vi "main.vi"() -> ()   [LabVIEW 2020]
doc: "This VI simulates the heat propagation and in/out flow in a square tank.\n\nThe heat propagation model used is a 2D rectangular heat wave PDE model to approximate the propagation of the heat in the liquid inside the tank. A heater is considered at the center of the base of the tank with set width and controllable output power. The walls of the tank are considered perfectly isolated. The heat losses are calculated by conduction from the surface of the liquid, through the air, to the outside (at room temperature).\n\nThe volume flow is controlled through the matrix that simulates the liquid for the PDE, that is, when enough volume is to be added to the tank, we add another row of points to the simulation (resp. remove for outward flow). Liquid is added at room temperature at the surface and removed from the bottom.\n\nThe transducers and actuators are modelled in this VI in such a way that the On/Off controller for the temperature (between EH 01 and TI 05) simulates a controller in a real plant. Room temperature is the only not-sensed-nor-actuated available variable to be used as noise. The tank graph should not be visible as well, but it makes the simulation much more pleasant to the eyes."
uses:
  TankResolution.ctl
  Heater.ctl
  <vilib>/Utility/error.llb/DialogType.ctl
panel:
  in  "temp_set_point":dbl(slide)=298.15 scale=0.0..100.0
  in  "temp_control":bool
  out "level_show":dbl format="%_3g m"
  out "temp_show_05":dbl format="%_3g ºC"
  out "temp_show_04":dbl format="%_3g ºC"
  out "temp_show_03":dbl format="%_3g ºC"
  out "temp_show_02":dbl format="%_3g ºC"
  out "temp_show_01":dbl format="%_3g ºC"
  out "termometer_05":dbl(slide) scale=0.0..100.0
  out "termometer_04":dbl(slide) scale=0.0..100.0
  out "termometer_03":dbl(slide) scale=0.0..100.0
  out "termometer_02":dbl(slide) scale=0.0..100.0
  out "termometer_01":dbl(slide) scale=0.0..100.0
  in  "BV 02":dbl(knob) scale=0.0..5.0
  in  "BV 01":dbl(knob) scale=0.0..5.0
  in  "EH 01":bool
  out "LI 01":dbl
  out "water_level":dbl
  out "TI 05":dbl
  out "TI 04":dbl
  out "TI 03":dbl
  out "TI 02":dbl
  out "TI 01":dbl
  out "temp_5":dbl
  out "temp_4":dbl
  out "temp_3":dbl
  out "temp_2":dbl
  out "temp_1":dbl
  out "out_flow (m^3/s)":dbl(knob) min=0.0 max=0.5 scale=0.0..0.01
  out "in_flow (m^3/s)":dbl(knob) min=0.0 max=0.5 scale=0.0..0.01
  in  "room_temperature":dbl(slide)=298.15 scale=273.15..373.15
  in  "heater":dbl(knob) scale=0.0..50.0
  in  "stop":bool
  out "PDE Plot":dbl[][](graph)
  # "Tank Model"
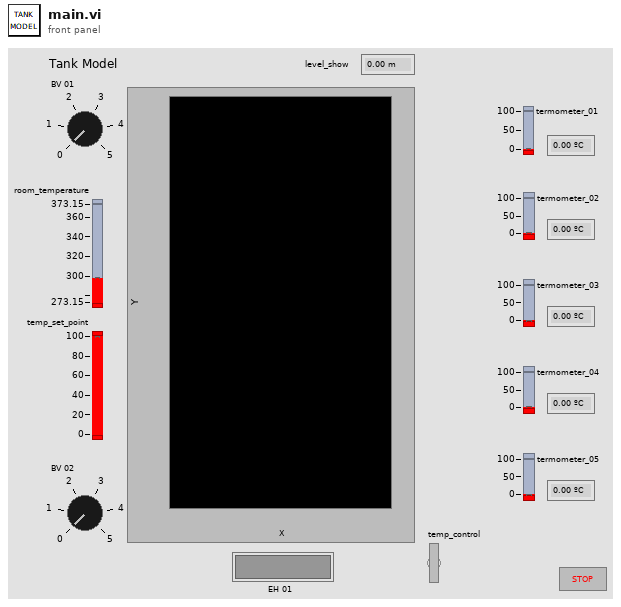
[diagram p1: front panel]
types:
  T1 = typedef "TankResolution.ctl" = cluster{"y_points_per_meter":i32, "x_points_per_meter":i32, "n_t_points":i32, "tank_height":dbl, "tank_width":dbl, "t_length_ms":u32}
  T2 = typedef "Liquid.ctl" = cluster{"liquid_temperature":dbl[][], "water_level":dbl, "room_temperature":dbl}
  T3 = typedef "DialogType.ctl" = u16
  T4 = typedef "Heater.ctl" = cluster{"heater_width":dbl, "heater_heat":dbl}
  T5 = typedef "LVOffsetAndMultiplierTypeDef.ctl" = cluster{"Offset":dbl, "Multiplier":dbl}
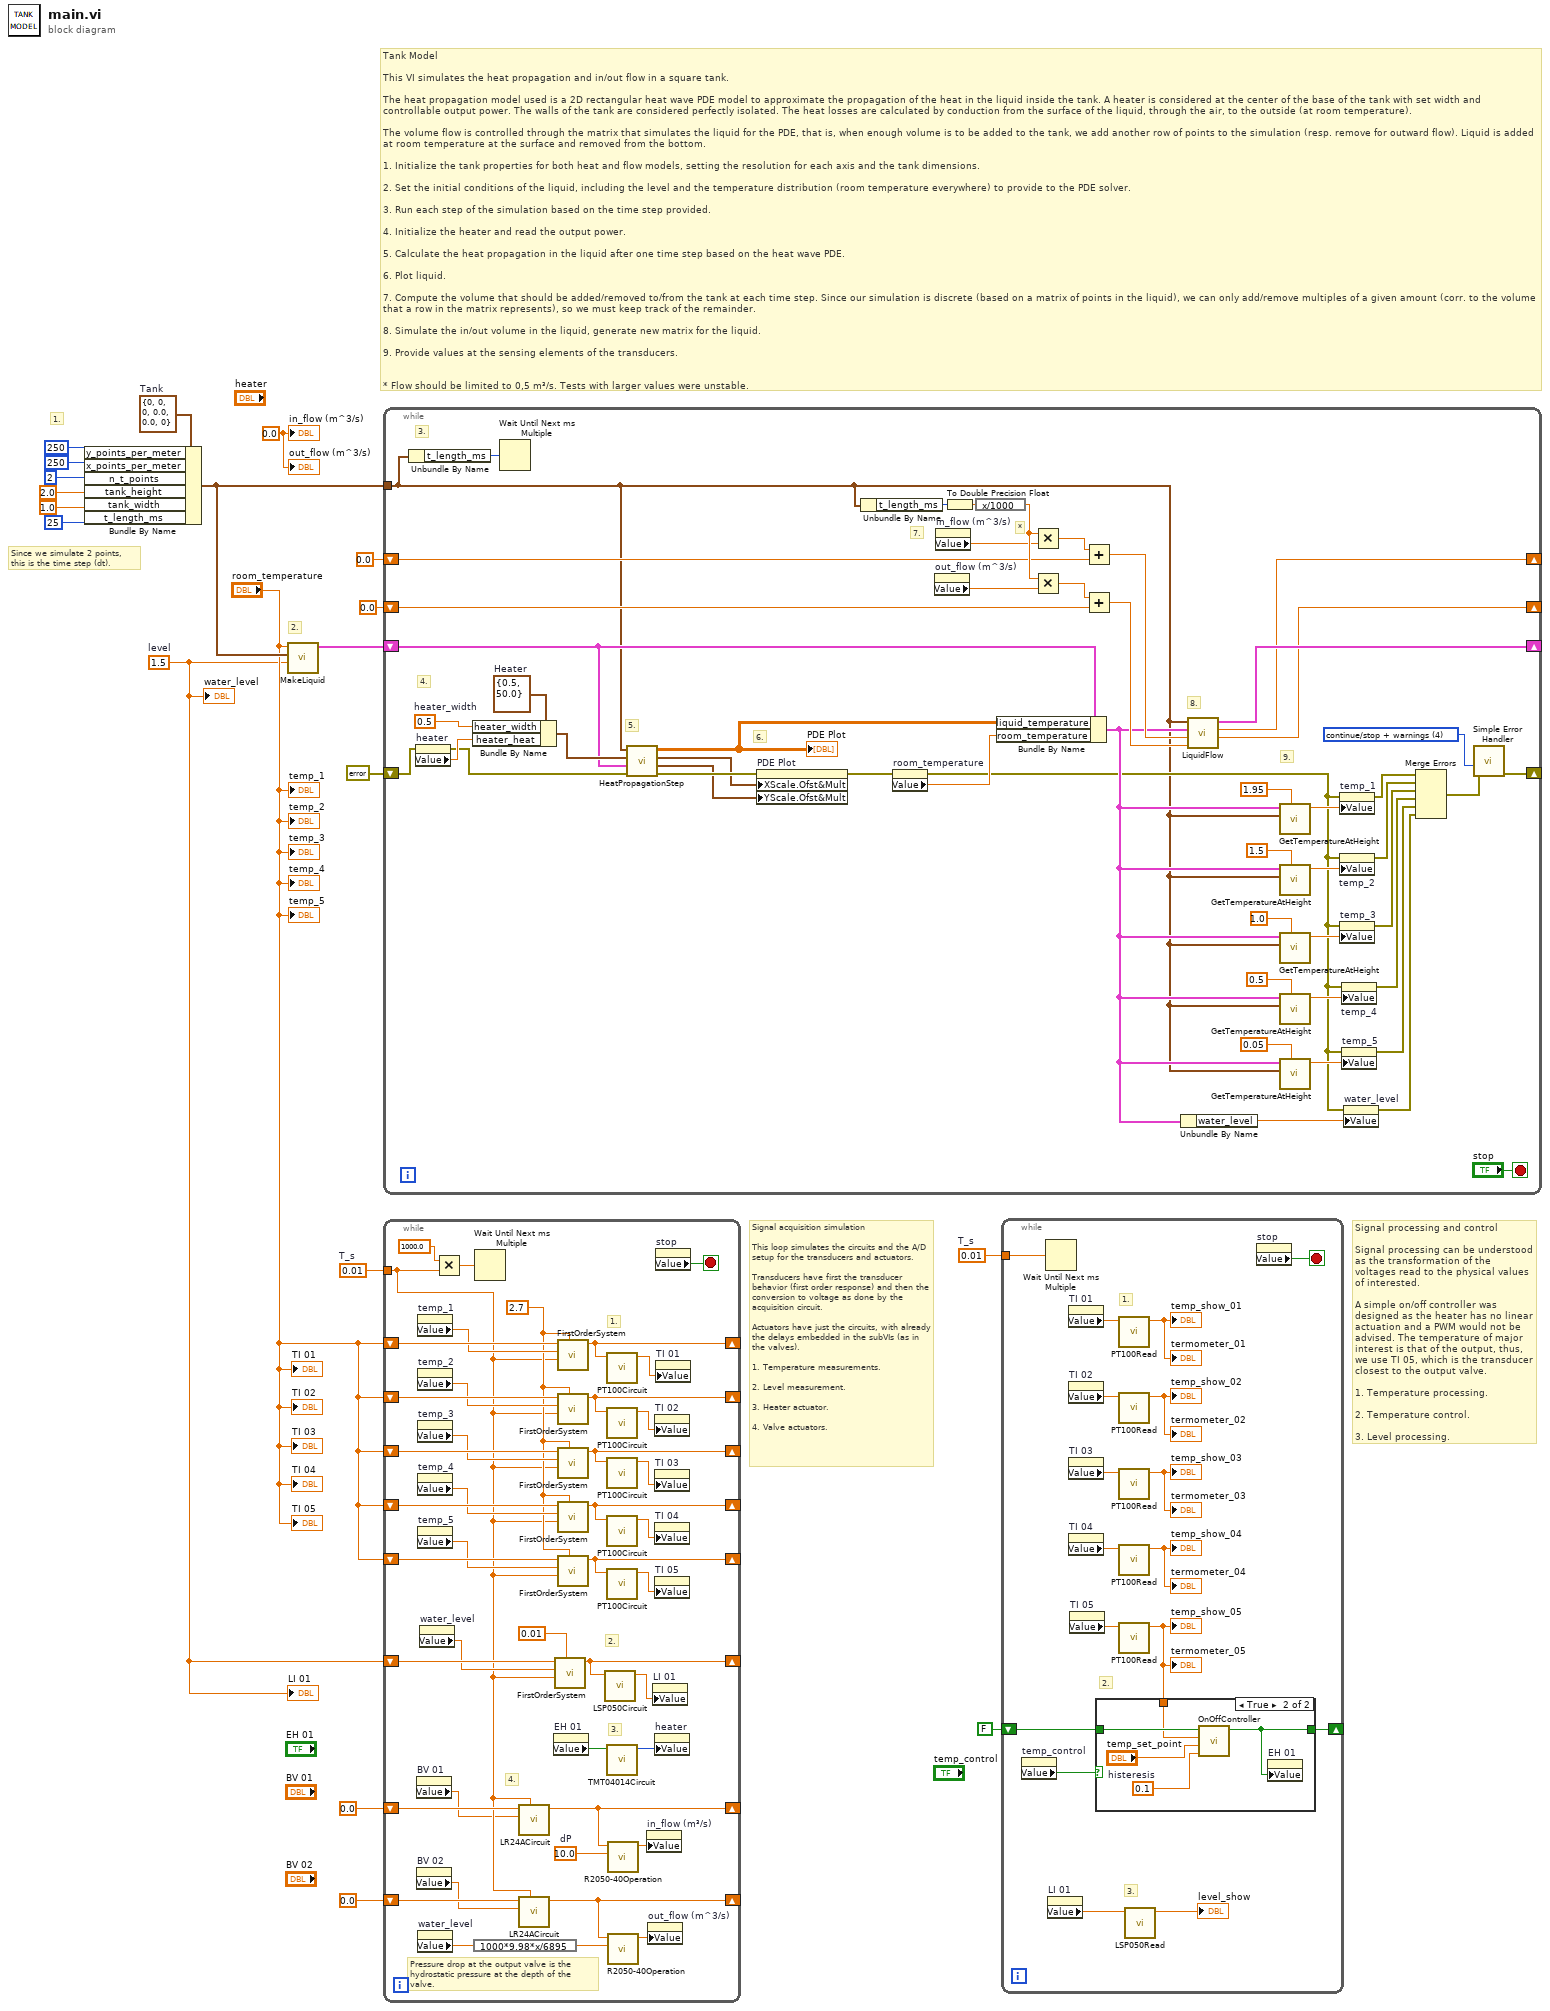
[diagram p0: block diagram]
diagram:
  w2 = 0.01  # T_s
  w5 = 0.0 ("in_flow (m")
  w8 = 0.01  # T_s
  w6 = 1.5  # level
  w20 = T1 {"y_points_per_meter"=0, "x_points_per_meter"=0, "n_t_points"=0, "tank_height"=0.0, "tank_width"=0.0, "t_length_ms"=0}  # Tank
  # "Signal processing and control\n\nSignal processing can be understood as the transformation of the voltages read to the physical values of interested.\n\nA simple on/off controller was designed as the heater has no linear actuation and a PWM would not be advised. The temperature of major interest is that of the output, thus, we use TI 05, which is the transducer closest to the output valve.\n\n1. Temperature processing.\n\n2. Temperature control.\n\n3. Level processing."
  # "Signal acquisition simulation\n\nThis loop simulates the circuits and the A/D setup for the transducers and actuators.\n\nTransducers have first the transducer behavior (first order response) and then the conversion to voltage as done by the acquisition circuit.\n\nActuators have just the circuits, with already the delays embedded in the subVIs (as in the valves).\n\n1. Temperature measurements.\n\n2. Level measurement.\n\n3. Heater actuator.\n\n4. Valve actuators."
  # "1."
  # "Tank Model\n\nThis VI simulates the heat propagation and in/out flow in a square tank.\n\nThe heat propagation model used is a 2D rectangular heat wave PDE model to approximate the propagation of the heat in the liquid inside the tank. A heater is considered at the center of the base of the tank with set width and controllable output power. The walls of the tank are considered perfectly isolated. The heat losses are calculated by conduction from the surface of the liquid, through the air, to the outside (at room temperature).\n\nThe volume flow is controlled through the matrix that simulates the liquid for the PDE, that is, when enough volume is to be added to the tank, we add another row of points to the simulation (resp. remove for outward flow). Liquid is added at room temperature at the surface and removed from the bottom.\n\n1. Initialize the tank properties for both heat and flow models, setting the resolution for each axis and the tank dimensions.\n\n2. Set the initial conditions of the liquid, including the level and the temperature distribution (room temperature everywhere) to provide to the PDE solver.\n\n3. Run each step of the simulation based on the time step provided.\n\n4. Initialize the heater and read the output power.\n\n5. Calculate the heat propagation in the liquid after one time step based on the heat wave PDE.\n\n6. Plot liquid.\n\n7. Compute the volume that should be added/removed to/from the tank at each time step. Since our simulation is discrete (based on a matrix of points in the liquid), we can only add/remove multiples of a given amount (corr. to the volume that a row in the matrix represents), so we must keep track of the remainder.\n\n8. Simulate the in/out volume in the liquid, generate new matrix for the liquid.\n\n9. Provide values at the sensing elements of the transducers.\n\n\n* Flow should be limited to 0,5 m³/s. Tests with larger values were unstable."
  # "2."
  # "Since we simulate 2 points,\nthis is the time step (dt)."
  n1 = Bundle By Name(cluster=w20, "y_points_per_meter"=250 ("n_y_points"), "x_points_per_meter"=250 ("x_resolution"), "n_t_points"=2, "tank_height"=2.0 ("y_length"), "tank_width"=1.0 ("x_length"), "t_length_ms"=u32 25) -> (w13:T1)
  n2 = call "MakeLiquid.vi"("level"=w6, "tank"=w13, "room_temperature"="room_temperature") -> ("liquid"=w12:T2)  [unwired: 8 in]
  n3 = while {
    tunnel: w13 -> [w21]
    shift-right: [w55] -> _
    shift-left: errorcluster {"status"=FALSE, "code"=0, "source"=""} ("error out") -> [w25]
    shift-right: [w50] -> _
    shift-left: w12 -> [w53]
    shift-right: [w49] -> _
    shift-left: 0.0 ("cumm_in_flow") -> [w56]
    shift-right: [w48] -> _
    shift-left: 0.0 ("cumm_out_flow") -> [w57]
    stop <- "stop" stop-if-true
    w54 = T3 4 items=["no dialog", "OK message", "continue or stop message", "OK message + warnings", "continue/stop + warnings"] ("type of dialog (OK msg:1)")
    w67 = T4 {"heater_width"=0.5, "heater_heat"=50.0}  # Heater
    w68 = 0.5  # heater_width
    # "9."
    # "*"
    # "6."
    # "4."
    # "3."
    # "8."
    # "7."
    # "5."
    n4 = Unbundle By Name(w21) -> ("t_length_ms"=w58:u32)
    n5 = property on="heater" class="Knob (strict)"(error in=w25) -> (error out=w24:errorcluster, "Value"=w26:dbl)  [unwired: 1 in, 1 out]
    n6 = Bundle By Name(cluster=w67, "heater_width"=w68, "heater_heat"=w26) -> (w66:T4)
    n7 = Wait Until Next ms Multiple(millisecond multiple=w58) -> ()  [unwired: 1 out]
    n8 = call "HeatPropagationStep.vi"("error in (no error)"=w24, "liquid"=w53, "heater"=w66, "tank"=w21) -> ("error out"=w72:errorcluster, "Y Scale"=w70:T5, "X Scale"=w71:T5, "next_temperature"=w47:dbl[][])  [unwired: 3 in]
    "PDE Plot" <- w47
    n9 = property on="PDE Plot" class="IntGraph (strict)"(error in=w72, "XScale.Ofst&Mult"=w71, "YScale.Ofst&Mult"=w70) -> (error out=w65:errorcluster)  [unwired: 1 in, 1 out]
    n10 = Unbundle By Name(w21) -> ("t_length_ms"=w59:u32)
    n11 = property on="room_temperature" class="Slide (strict)"(error in=w65) -> (error out=w27:errorcluster, "Value"=w64:dbl)  [unwired: 1 in, 1 out]
    n12 = property on="out_flow (m^3/s)" class="Knob (strict)"() -> ("Value"=w22:dbl)  [unwired: 2 in, 2 out]
    n13 = property on="in_flow (m^3/s)" class="Knob (strict)"() -> ("Value"=w23:dbl)  [unwired: 2 in, 2 out]
    n14 = To Double Precision Float(number=w59) -> (double precision float=w60:dbl)
    n15 = expression code="x/1000"(w60) -> (w63:dbl)
    n16 = Bundle By Name(cluster=w53, "liquid_temperature"=w47, "room_temperature"=w64) -> (w30:T2)
    n17 = Multiply(x=w63, y=w23) -> (x*y=w62:dbl)
    n18 = Multiply(x=w63, y=w22) -> (x*y=w61:dbl)
    n19 = Add(x=w62, y=w56) -> (x+y=w52:dbl)
    n20 = Add(x=w61, y=w57) -> (x+y=w51:dbl)
    n21 = Unbundle By Name(w30) -> ("water_level"=w29:dbl)
    n22 = call "LiquidFlow.vi"("out_vol"=w51, "in_vol"=w52, "liquid"=w30, "tank"=w21) -> ("remainder_out_vol"=w48:dbl, "remainder_in_vol"=w49:dbl, "next_liquid"=w50:T2)  [unwired: 5 in]
    n23 = call "GetTemperatureAtHeight.vi"("height"=1.95 ("tank_height"), "tank"=w21, "liquid"=w30) -> ("temperature"=w46:dbl)  [unwired: 8 in]
    n24 = call "GetTemperatureAtHeight.vi"("height"=1.5 ("tank_height"), "tank"=w21, "liquid"=w30) -> ("temperature"=w37:dbl)  [unwired: 8 in]
    n25 = call "GetTemperatureAtHeight.vi"("height"=1.0 ("tank_height"), "tank"=w21, "liquid"=w30) -> ("temperature"=w38:dbl)  [unwired: 8 in]
    n26 = call "GetTemperatureAtHeight.vi"("height"=0.5 ("tank_height"), "tank"=w21, "liquid"=w30) -> ("temperature"=w39:dbl)  [unwired: 8 in]
    n27 = call "GetTemperatureAtHeight.vi"("height"=0.05 ("tank_height"), "tank"=w21, "liquid"=w30) -> ("temperature"=w40:dbl)  [unwired: 8 in]
    n28 = property on="temp_1" class="DigNum (strict)"(error in=w27, "Value"=w46) -> (error out=w35:errorcluster)  [unwired: 1 in, 1 out]
    n29 = property on="temp_2" class="DigNum (strict)"(error in=w27, "Value"=w37) -> (error out=w34:errorcluster)  [unwired: 1 in, 1 out]
    n30 = property on="temp_3" class="DigNum (strict)"(error in=w27, "Value"=w38) -> (error out=w32:errorcluster)  [unwired: 1 in, 1 out]
    n31 = property on="temp_4" class="DigNum (strict)"(error in=w27, "Value"=w39) -> (error out=w31:errorcluster)  [unwired: 1 in, 1 out]
    n32 = property on="temp_5" class="DigNum (strict)"(error in=w27, "Value"=w40) -> (error out=w33:errorcluster)  [unwired: 1 in, 1 out]
    n33 = property on="water_level" class="DigNum (strict)"(error in=w27, "Value"=w29) -> (error out=w28:errorcluster)  [unwired: 1 in, 1 out]
    n34 = Merge Errors(w35, w34, w32, w31, w33, w28) -> (w36:errorcluster)
    n35 = call <vilib>:"Simple Error Handler.vi"("type of dialog (OK msg:1)"=w54, "error in (no error)"=w36) -> ("error out"=w55:errorcluster)  [unwired: 3 in, 4 out]
  }
  n36 = while {
    tunnel: w8 -> [w81]
    shift-right: [w101] -> _
    shift-left: "room_temperature" -> [w114]
    shift-right: [w99] -> _
    shift-left: "room_temperature" -> [w111]
    shift-right: [w98] -> _
    shift-left: "room_temperature" -> [w112]
    shift-right: [w97] -> _
    shift-left: "room_temperature" -> [w110]
    shift-right: [w96] -> _
    shift-left: "room_temperature" -> [w109]
    shift-right: [w88] -> _
    shift-left: w6 -> [w91]
    shift-right: [w83] -> _
    shift-left: 0.0 ("angle") -> [w84]
    shift-right: [w80] -> _
    shift-left: 0.0 ("angle") -> [w79]
    stop <- w115 stop-if-true
    w82 = 10.0  # dP
    w104 = 2.7 ("T")
    # "Pressure drop at the output valve is the hydrostatic pressure at the depth of the valve."
    # "4."
    # "3."
    # "2."
    # "1."
    n37 = property on="BV 01" class="Knob (strict)"() -> ("Value"=w74:dbl)  [unwired: 2 in, 2 out]
    n38 = property on="BV 02" class="Knob (strict)"() -> ("Value"=w73:dbl)  [unwired: 2 in, 2 out]
    n39 = property on="temp_1" class="DigNum (strict)"() -> ("Value"=w113:dbl)  [unwired: 2 in, 2 out]
    n40 = property on="temp_2" class="DigNum (strict)"() -> ("Value"=w108:dbl)  [unwired: 2 in, 2 out]
    n41 = property on="temp_3" class="DigNum (strict)"() -> ("Value"=w107:dbl)  [unwired: 2 in, 2 out]
    n42 = property on="temp_4" class="DigNum (strict)"() -> ("Value"=w106:dbl)  [unwired: 2 in, 2 out]
    n43 = property on="temp_5" class="DigNum (strict)"() -> ("Value"=w105:dbl)  [unwired: 2 in, 2 out]
    n44 = property on="water_level" class="DigNum (strict)"() -> ("Value"=w78:dbl)  [unwired: 2 in, 2 out]
    n45 = property on="water_level" class="DigNum (strict)"() -> ("Value"=w89:dbl)  [unwired: 2 in, 2 out]
    n46 = Multiply(x=1000.0, y=w81) -> (x*y=w103:dbl)
    n47 = expression code="1000*9.98*x/6895"(w78) -> (w77:dbl)
    n48 = Wait Until Next ms Multiple(millisecond multiple=w103) -> ()  [unwired: 1 out]
    n49 = call "LR24ACircuit.vi"("dt"=w81, "voltage"=w74, "curr_angle"=w84) -> ("angle"=w83:dbl)  [unwired: 8 in]
    n50 = call "LR24ACircuit.vi"("dt"=w81, "voltage"=w73, "curr_angle"=w79) -> ("angle"=w80:dbl)  [unwired: 8 in]
    n51 = property on="EH 01" class="Bool (strict)"() -> ("Value"=w75:bool)  [unwired: 2 in, 2 out]
    n52 = call "FirstOrderSystem.vi"("T"=0.01, "T_s"=w81, "u_k-1"=w89, "y_k-1"=w91) -> ("y_k"=w88:dbl)  [unwired: 7 in]
    n53 = call "FirstOrderSystem.vi"("T"=w104, "T_s"=w81, "u_k-1"=w113, "y_k-1"=w114) -> ("y_k"=w101:dbl)  [unwired: 7 in]
    n54 = call "FirstOrderSystem.vi"("T"=w104, "T_s"=w81, "u_k-1"=w108, "y_k-1"=w111) -> ("y_k"=w99:dbl)  [unwired: 7 in]
    n55 = call "FirstOrderSystem.vi"("T"=w104, "T_s"=w81, "u_k-1"=w107, "y_k-1"=w112) -> ("y_k"=w98:dbl)  [unwired: 7 in]
    n56 = call "FirstOrderSystem.vi"("T"=w104, "T_s"=w81, "u_k-1"=w106, "y_k-1"=w110) -> ("y_k"=w97:dbl)  [unwired: 7 in]
    n57 = call "FirstOrderSystem.vi"("T"=w104, "T_s"=w81, "u_k-1"=w105, "y_k-1"=w109) -> ("y_k"=w96:dbl)  [unwired: 7 in]
    n58 = call "LSP050Circuit.vi"("water_level"=w88) -> ("voltage"=w87:dbl)  [unwired: 10 in]
    n59 = call "PT100Circuit.vi"("temp"=w101) -> ("voltage"=w100:dbl)  [unwired: 10 in]
    n60 = call "PT100Circuit.vi"("temp"=w99) -> ("voltage"=w95:dbl)  [unwired: 10 in]
    n61 = call "PT100Circuit.vi"("temp"=w98) -> ("voltage"=w94:dbl)  [unwired: 10 in]
    n62 = call "PT100Circuit.vi"("temp"=w97) -> ("voltage"=w93:dbl)  [unwired: 10 in]
    n63 = call "PT100Circuit.vi"("temp"=w96) -> ("voltage"=w92:dbl)  [unwired: 10 in]
    n64 = call "TMT04014Circuit.vi"("power_heater?"=w75) -> ("heater_output"=w86:i16)  [unwired: 10 in]
    n65 = call "R2050-40Operation.vi"("pressure_drop (psia)"=w82, "angle (deg)"=w83) -> ("flow (m³/s)"=w85:dbl)  [unwired: 9 in]
    n66 = call "R2050-40Operation.vi"("pressure_drop (psia)"=w77, "angle (deg)"=w80) -> ("flow (m³/s)"=w76:dbl)  [unwired: 9 in]
    n67 = property on="in_flow (m³/s)" class="Knob (strict)"("Value"=w85) -> ()  [unwired: 2 in, 2 out]
    n68 = property on="out_flow (m^3/s)" class="Knob (strict)"("Value"=w76) -> ()  [unwired: 2 in, 2 out]
    n69 = property on="LI 01" class="DigNum (strict)"("Value"=w87) -> ()  [unwired: 2 in, 2 out]
    n70 = property on="TI 02" class="DigNum (strict)"("Value"=w95) -> ()  [unwired: 2 in, 2 out]
    n71 = property on="TI 03" class="DigNum (strict)"("Value"=w94) -> ()  [unwired: 2 in, 2 out]
    n72 = property on="TI 04" class="DigNum (strict)"("Value"=w93) -> ()  [unwired: 2 in, 2 out]
    n73 = property on="TI 05" class="DigNum (strict)"("Value"=w92) -> ()  [unwired: 2 in, 2 out]
    n74 = property on="heater" class="Knob (strict)"("Value"=w86) -> ()  [unwired: 2 in, 2 out]
    n75 = property on="stop" class="Bool (strict)"() -> ("Value"=w115:bool)  [unwired: 2 in, 2 out]
    n76 = property on="TI 01" class="DigNum (strict)"("Value"=w100) -> ()  [unwired: 2 in, 2 out]
  }
  n77 = while {
    tunnel: w2 -> [w132]
    shift-right: [w128] -> _
    shift-left: FALSE ("u_k") -> [w130]
    stop <- w129 stop-if-true
    # "3."
    # "2."
    # "1."
    n78 = property on="temp_control" class="Bool (strict)"() -> ("Value"=w116:bool)  [unwired: 2 in, 2 out]
    n79 = Wait Until Next ms Multiple(millisecond multiple=w132) -> ()  [unwired: 1 out]
    n80 = property on="LI 01" class="DigNum (strict)"() -> ("Value"=w117:dbl)  [unwired: 2 in, 2 out]
    n81 = property on="TI 01" class="DigNum (strict)"() -> ("Value"=w127:dbl)  [unwired: 2 in, 2 out]
    n82 = property on="TI 02" class="DigNum (strict)"() -> ("Value"=w125:dbl)  [unwired: 2 in, 2 out]
    n83 = property on="TI 03" class="DigNum (strict)"() -> ("Value"=w124:dbl)  [unwired: 2 in, 2 out]
    n84 = property on="TI 04" class="DigNum (strict)"() -> ("Value"=w123:dbl)  [unwired: 2 in, 2 out]
    n85 = property on="TI 05" class="DigNum (strict)"() -> ("Value"=w131:dbl)  [unwired: 2 in, 2 out]
    n86 = call "PT100Read.vi"("TI XX"=w127) -> ("temp"=→"termometer_01" →"temp_show_01":dbl)  [unwired: 10 in]
    n87 = call "PT100Read.vi"("TI XX"=w125) -> ("temp"=→"temp_show_02" →"termometer_02":dbl)  [unwired: 10 in]
    n88 = call "PT100Read.vi"("TI XX"=w124) -> ("temp"=→"temp_show_03" →"termometer_03":dbl)  [unwired: 10 in]
    n89 = call "PT100Read.vi"("TI XX"=w123) -> ("temp"=→"temp_show_04" →"termometer_04":dbl)  [unwired: 10 in]
    n90 = call "PT100Read.vi"("TI XX"=w131) -> ("temp"=w119:dbl)  [unwired: 10 in]
    "temp_show_05" <- w119
    "termometer_05" <- w119
    n91 = case shown="True" w116 {
      tunnel: w130 -> [w133 w138]
      tunnel: [w133 w136] -> w128
      tunnel: w119 -> [_ w135]
      frame False {
      }
      frame True {
        w137 = 0.1  # histeresis
        n92 = call "OnOffController.vi"("histeresis"=w137, "set_point"="temp_set_point", "temp"=w135, "u_k-1"=w138) -> ("u_k"=w136:bool)  [unwired: 7 in]
        n93 = property on="EH 01" class="Bool (strict)"("Value"=w136) -> ()  [unwired: 2 in, 2 out]
      }
    }
    n94 = call "LSP050Read.vi"("voltage"=w117) -> ("level"=→"level_show":dbl)  [unwired: 10 in]
    n95 = property on="stop" class="Bool (strict)"() -> ("Value"=w129:bool)  [unwired: 2 in, 2 out]
  }
  "temp_1" <- "room_temperature"
  "temp_2" <- "room_temperature"
  "temp_3" <- "room_temperature"
  "temp_4" <- "room_temperature"
  "temp_5" <- "room_temperature"
  "TI 01" <- "room_temperature"
  "TI 02" <- "room_temperature"
  "TI 03" <- "room_temperature"
  "TI 04" <- "room_temperature"
  "TI 05" <- "room_temperature"
  "water_level" <- w6
  "LI 01" <- w6
  "in_flow (m^3/s)" <- w5
  "out_flow (m^3/s)" <- w5
